vi "Curtin1_ReadWfm.vi"(11 "appended path":path) -> (0 "error out":errorcluster, 2 "all waveforms in record":waveform(dbl)[](array[waveform]))   [LabVIEW 2022 SP3]
uses:
  <vilib>/Waveform/WDTFileIO.llb/Read Waveform from File.vi
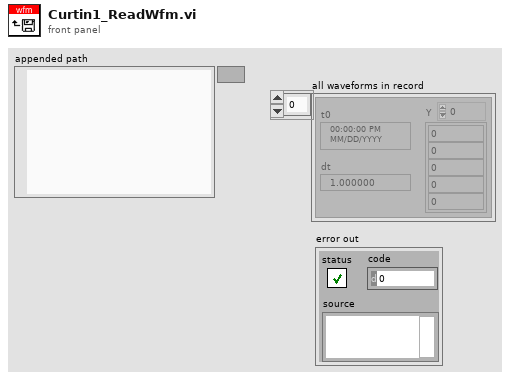
[diagram p1: front panel]
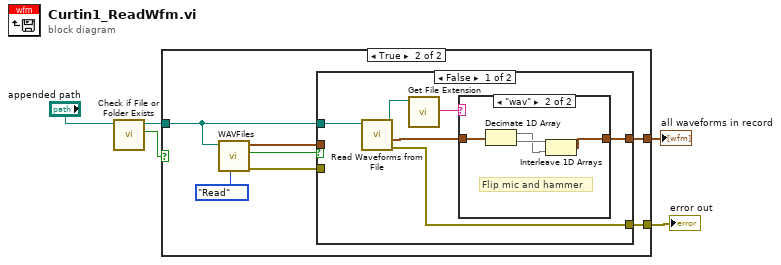
[diagram p0: block diagram]
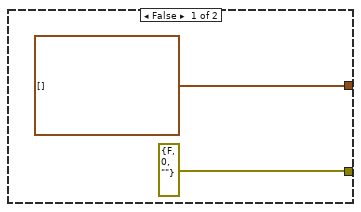
[diagram p2: hidden frame]
diagram:
  n1 = call <vilib>:"Check if File or Folder Exists.vi"("path"="appended path") -> ("file or folder exists?"=w2:bool)  [unwired: 8 in, 2 out]
  n2 = case shown="True" w2 {
    tunnel: [waveform(dbl)[] [] ("all waveforms in record") w13] -> w4
    tunnel: "appended path" -> [_ w11]
    tunnel: [errorcluster {"status"=FALSE, "code"=0, "source"=""} ("error out") w12] -> w1
    frame False {
    }
    frame True {
      n3 = call "WAVFiles.vi"("Task"=enum16{"Read", "Write", "wfm"}."Read", "WAV File"=w11) -> ("error out"=w8:errorcluster, "Valid?"=w10:bool, "Data"=w9:waveform(dbl)[])  [unwired: 6 in, 1 out]
      n4 = case shown="False" w10 {
        tunnel: [w17 w26] -> w13
        tunnel: [w15 w25] -> w12
        tunnel: w11 -> [w14 _]
        tunnel: w9 -> [_ w26]
        tunnel: w8 -> [_ w25]
        frame False {
          n5 = call-poly <vilib>:"Read Waveforms from File.vi"("file path (dialog if empty)"=w14) -> ("error out"=w15:errorcluster, "all waveforms in record"=w16:waveform(dbl)[], "new file path (Not A Path if cancelled)"=w19:path)  [unwired: 5 in, 1 out]
          n6 = call <vilib>:"Get File Extension.vi"("file"=w19) -> ("lowercase file extension"=w18:string)  [unwired: 6 in, 4 out]
          n7 = case shown="\"wav\"" w18 {
            tunnel: [w20 w21] -> w17
            tunnel: w16 -> [w20 w22]
            frame Default {
            }
            frame "wav" {
              # "Flip mic and hammer"
              n8 = Decimate 1D Array(w22) -> (w23:waveform(dbl)[], w24:waveform(dbl)[])
              n9 = Interleave 1D Arrays(w24, w23) -> (w21:waveform(dbl)[])
            }
          }
        }
        frame True {
        }
      }
    }
  }
  "all waveforms in record" <- w4
  "error out" <- w1
